vi "NumericalDerivative-of-3ds.vi"() -> ()   [LabVIEW 2021, in "Nanonis Prog Interface.lvlib"]
uses:
  Nanonis Prog Interface.lvlib
  <vilib>/Analysis/NI_AALPro.lvlib
panel:
  out "error out Write file":errorcluster
  out "error out Read file":errorcluster
  in  "Fit length for derivative":u16=2 min=2 max=1000
  in  "Binary Spectroscopy File":path
  # "This VI takes a 3ds file as input to create a new 3ds file with the derived signals.\nIf the source files contains I/V curves this VI will create a new file containing calculated dI/dV curves.\nThe derivative is calculated by determining the slope of a piece-wise linear fit to the input signals. Due to the nature of this derivative some points at the beginning and at the end will be cut, so the resulting curves will have less points and the sweep signal limits will be different."
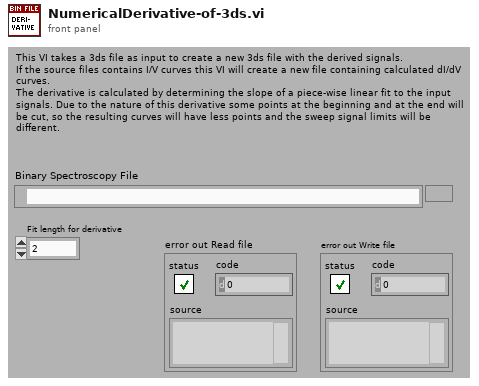
[diagram p1: front panel]
types:
  T1 = typedef "Nanonis Prog Interface.lvlib/Binary_SpectroscopyFile-Config.ctl" = cluster{"Num Par":i32, "Exp size":i32, "Points":i32, "Grid Dim X":i32, "Grid Dim Y":i32, "Header size":i32, "Channels":string[], "Parameters":string[], "Sweep Signal":string, "Grid":cluster{"center X (m)":sgl, "center Y (m)":sgl, "width (m)":sgl, "height (m)":sgl, "angle (deg)":sgl}}
  T2 = cluster{"center X (m)":sgl, "center Y (m)":sgl, "width (m)":sgl, "height (m)":sgl, "angle (deg)":sgl}
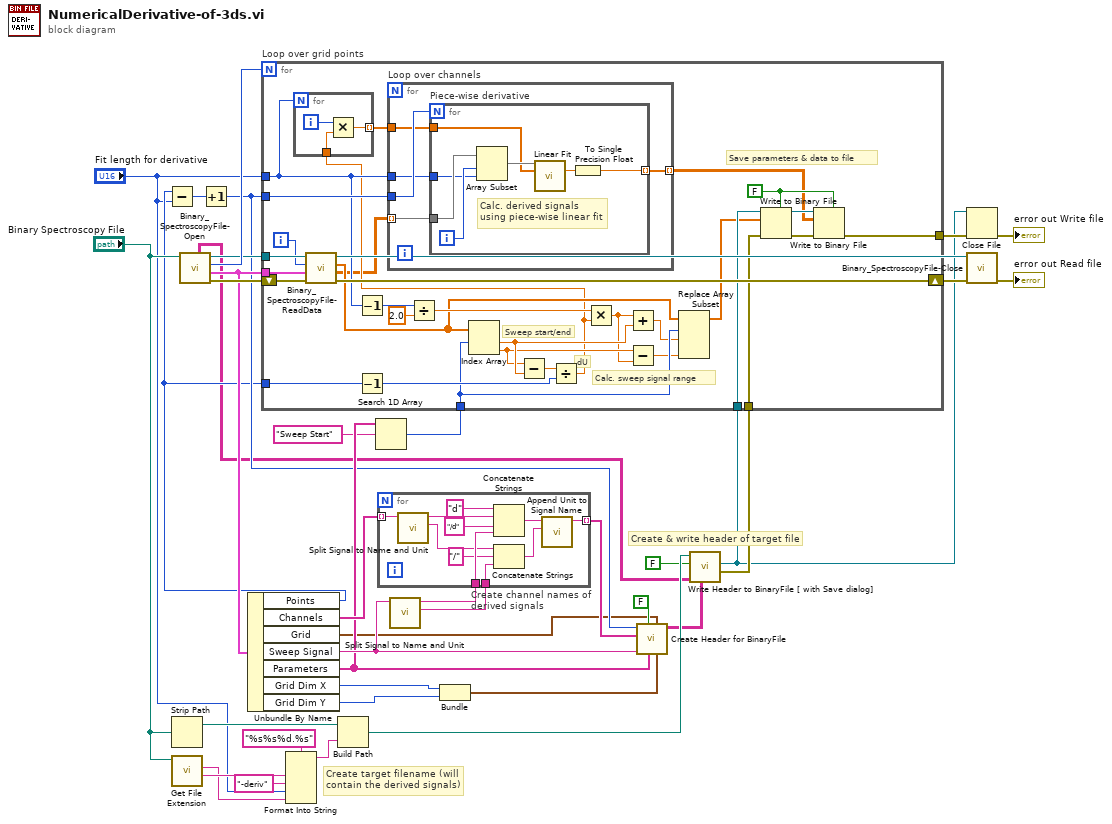
[diagram p0: block diagram]
diagram:
  # "Create & write header of target file"
  # "Create target filename (will contain the derived signals)"
  n1 = Strip Path(path="Binary Spectroscopy File") -> (stripped path=w31:path)  [unwired: 1 out]
  n2 = call <vilib>:"Get File Extension.vi"("file"="Binary Spectroscopy File") -> ("filename without extension"=w4:string, "lowercase file extension"=w3:string)  [unwired: 6 in, 3 out]
  n3 = call "Binary_SpectroscopyFile-Open.vi"("Binary Spectroscopy File"="Binary Spectroscopy File") -> ("error out"=w37:errorcluster, "Config"=w25:T1, "Number of Experiments"=w38:i32, "File ref"=w26:refnum<file>, "Global Attributes"=w7:string[][])  [unwired: 6 in]
  n4 = Unbundle By Name(w25) -> ("Points"=w14:i32, "Channels"=w24:string[], "Grid"=w13:T2, "Sweep Signal"=w23:string, "Parameters"=w18:string[], "Grid Dim X"=w35:i32, "Grid Dim Y"=w34:i32)
  n5 = Subtract(x=w14, y="Fit length for derivative") -> (x-y=w19:i32)
  n6 = Increment(x=w19) -> (x+1=w15:i32)
  n7 = Format Into String(format string="%s%s%d.%s", w4, "-deriv" ("string"), "Fit length for derivative", w3) -> (resulting string=w2:string)  [unwired: 2 in, 1 out]
  n8 = Build Path(base path=w31, name or relative path=w2) -> (appended path=w30:path)
  n9 = Search 1D Array(1D array=w18, element="Sweep Start") -> (index of element=w16:i32)  [unwired: 1 in]
  n10 = call <userlib>:"Split Signal to Name and Unit.vi"("Name with unit"=w23) -> ("Unit"=w21:string, "Name"=w22:string)  [unwired: 5 in]
  n11 = for "Create channel names of derived signals" {
    tunnel: w24 -> [w49] mode=indexing
    tunnel: w22 -> [w45]
    tunnel: w21 -> [w42]
    tunnel: [w39] -> w20 mode=indexing
    n12 = call <userlib>:"Split Signal to Name and Unit.vi"("Name with unit"=w49) -> ("Unit"=w44:string, "Name"=w48:string)  [unwired: 5 in]
    n13 = Concatenate Strings("d" ("string"), w48, "/d" ("string"), w45) -> (w41:string)
    n14 = Concatenate Strings(w44, "/" ("string"), w42) -> (w40:string)
    n15 = call <userlib>:"Append Unit to Signal Name.vi"("Unit"=w40, "Name"=w41) -> ("Name with unit"=w39:string)  [unwired: 5 in]
  }
  n16 = Bundle("Grid Dim X"=w35, "Grid Dim Y"=w34) -> (w33:cluster{"Grid Dim X":i32, "Grid Dim Y":i32})  [unwired: 1 in]
  n17 = call <userlib>:"Create Header for BinaryFile.vi"("Grid points"=w33, "Grid param"=w13, "Fixed parameters"=w18, "Backward sweep"=FALSE, "Sweep signal"=w23, "Channels"=w20, "Points per sweep"=w15) -> ("Header (fixed attributes)"=w28:string[][])  [unwired: 4 in]
  n18 = call <userlib>:"Write Header to BinaryFile [ with Save dialog].vi"("Fixed Attributes"=w28, "Attributes in"=w7, "Show Dialog? (T)"=FALSE, "Filename"=w30) -> ("Error out"=w12:errorcluster, "File ref"=w10:refnum<file>)  [unwired: 4 in, 2 out]
  n19 = for "Loop over grid points" {
    N: w38 -> [_]
    tunnel: w26 -> [w80]
    tunnel: w25 -> [w78]
    shift-right: [w76] -> w27
    shift-left: w37 -> [w77]
    tunnel: w10 -> [w58]
    tunnel: "Fit length for derivative" -> [w61]
    tunnel: w16 -> [w65]
    tunnel: w14 -> [w75]
    tunnel: w15 -> [w62]
    tunnel: w12 -> [w56]
    tunnel: [w50] -> w11
    i -> [w79]
    w54 = FALSE ("prepend array or string size? (T)")
    # "dU"
    # "Sweep start/end"
    # "Save parameters & data to file"
    # "Calc. sweep signal range"
    n20 = call "Binary_SpectroscopyFile-ReadData.vi"("error in"=w77, "Config"=w78, "Experiment to read (Index)"=w79, "File ref In"=w80) -> ("error out"=w76:errorcluster, "data"=w52:sgl[][], "Parameter values"=w66:sgl[])  [unwired: 4 in, 1 out]
    n21 = Decrement(x=w61) -> (x-1=w72:u16)
    n22 = Decrement(x=w75) -> (x-1=w74:i32)
    n23 = Divide(x=w72, y=sgl 2.0) -> (x/y=w70:sgl)
    n24 = Index Array(array=w66, index #1=w65) -> (element #1=w69:sgl, element #2=w68:sgl)  [unwired: 1 in]
    n25 = Subtract(x=w68, y=w69) -> (x-y=w73:sgl)
    n26 = Divide(x=w73, y=w74) -> (x/y=w60:sgl)
    n27 = for {
      N: w61 -> [_]
      tunnel: w60 -> [w82]
      tunnel: [w81] -> w59 mode=indexing
      i -> [w83]
      n28 = Multiply(x=w83, y=w82) -> (x*y=w81:sgl)
    }
    n29 = for "Loop over channels" {
      tunnel: w52 -> [w87] mode=indexing
      tunnel: w61 -> [w86]
      tunnel: w62 -> [w88]
      tunnel: w59 -> [w85]
      tunnel: [w84] -> w51 mode=indexing
      n30 = for "Piece-wise derivative" {
        N: w88 -> [_]
        tunnel: w87 -> [w95]
        tunnel: w86 -> [w93]
        tunnel: w85 -> [w91]
        tunnel: [w89] -> w84 mode=indexing
        i -> [w94]
        # "Calc. derived signals using piece-wise linear fit"
        n31 = Array Subset(array=w95, index=w94, length=w93) -> (w92:sgl[])
        n32 = call <vilib>:"Linear Fit.vi"("Y"=w92, "X"=w91) -> ("slope"=w90:dbl)  [unwired: 9 in, 4 out]
        n33 = To Single Precision Float(number=w90) -> (single precision float=w89:sgl)
      }
    }
    n34 = Multiply(x=w70, y=w60) -> (x*y=w67:sgl)
    n35 = Add(x=w67, y=w69) -> (x+y=w64:sgl)
    n36 = Subtract(x=w68, y=w67) -> (x-y=w63:sgl)
    n37 = Replace Array Subset(array=w66, new element #1=w64, index #1=w65, new element #2=w63) -> (w57:sgl[])  [unwired: 1 in]
    n38 = Write to Binary File(file (use dialog)=w58, data=w57, error in=w56, 5:w54) -> (refnum out=w55:refnum<file>, error out=w53:errorcluster)  [unwired: 2 in, 1 out]
    n39 = Write to Binary File(file (use dialog)=w55, data=w51, error in=w53, 5:w54) -> (error out=w50:errorcluster)  [unwired: 2 in, 2 out]
  }
  n40 = Close File(refnum=w10, error in=w11) -> (error out=→"error out Write file":errorcluster)  [unwired: 1 out]
  n41 = call "Binary_SpectroscopyFile-Close.vi"("error in"=w27, "File ref"=w26) -> ("error out"=→"error out Read file":errorcluster)  [unwired: 9 in]
